vi "Actor Core.vi"(8 "error in":cluster{"状态":bool, "代码":i32, "源":string} caption="错误输入", 11 "Beta":refnum<class "Beta.lvclass"> caption="DNL_Beta") -> (0 "error out":cluster{"状态":bool, "代码":i32, "源":string} caption="错误输出", 3 "操作者输出":refnum<class "Actor.lvclass">)   [LabVIEW 2013, in "Beta操作者.lvlib" / "Beta.lvclass"]
doc: "Actor Core.vi包含操作者的主要消息处理循环。操作者通常位于该循环中，在各种消息到达时对消息进行处理。如Do.vi消息返回任何错误，该循环将停止运行，错误代码43将被作为“无错误停止”的标准信号发送给调用方。如需更改上述行为，可在子孙类的Handle Error.vi中对该部分逻辑进行重写。"
uses:
  Beta.lvclass
  <vilib>/ActorFramework/Actor/Actor.lvclass
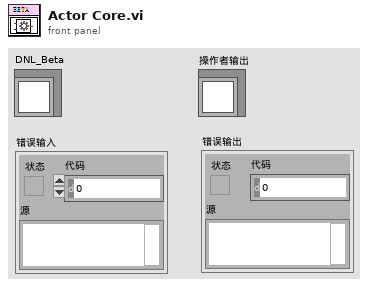
[diagram p1: front panel]
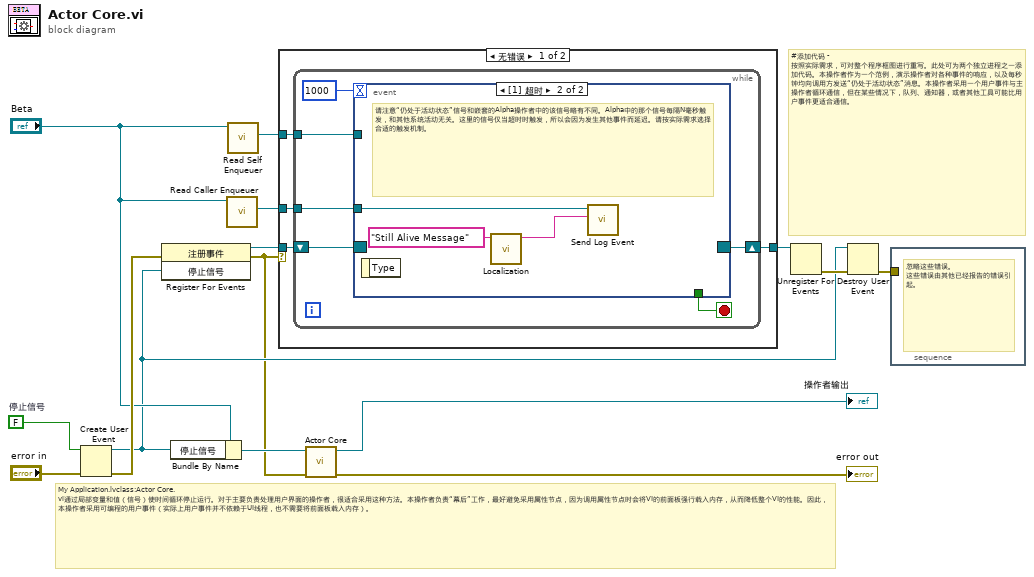
[diagram p0: block diagram]
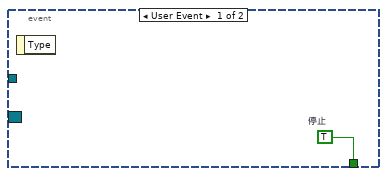
[diagram p2: hidden frame]
diagram:
  w11 = FALSE  # 停止信号
  # "My Application.lvclass:Actor Core.vi通过局部变量和值（信号）使时间循环停止运行。对于主要负责处理用户界面的操作者，很适合采用这种方法。本操作者负责“幕后”工作，最好避免采用属性节点，因为调用属性节点时会将VI的前面板强行载入内存，从而降低整个VI的性能。因此，本操作者采用可编程的用户事件（实际上用户事件并不依赖于UI线程，也不需要将前面板载入内存）。"
  # "#添加代码 - 按照实际需求，可对整个程序框图进行重写。此处可为两个独立进程之一添加代码。本操作者作为一个范例，演示操作者对各种事件的响应，以及每秒钟均向调用方发送“仍处于活动状态”消息。本操作者采用一个用户事件与主操作者循环通信，但在某些情况下，队列、通知器，或者其他工具可能比用户事件更适合通信。"
  n1 = Create User Event(user event datatype=w11, error in="error in") -> (user event=w4:refnum<user-event>, error out=w10:errorcluster)
  n2 = register-events(error in=w10, w4) -> (reference out=w9:refnum<event-registration>, error out=w2:errorcluster)  [unwired: 1 in]
  n3 = Bundle By Name(cluster="Beta", "停止信号"=w4) -> (w6:refnum<class "Beta.lvclass">)
  n4 = call <vilib>:"Read Caller Enqueuer.vi"("Actor"="Beta") -> ("Caller Enqueuer"=w13:refnum<class "Message Enqueuer.lvclass">)  [unwired: 10 in]
  n5 = call <vilib>:"Read Self Enqueuer.vi"("Actor"="Beta") -> ("Self Enqueuer"=w14:refnum<class "Message Enqueuer.lvclass">)  [unwired: 10 in]
  n6 = case shown="无错误" w2 {
    tunnel: w14 -> [w19 _]
    tunnel: w13 -> [w18 _]
    tunnel: w9 -> [w17 w30]
    tunnel: [w16 w30] -> w3
    frame No Error {
      n7 = while {
        tunnel: w19 -> [w24]
        tunnel: w18 -> [w23]
        shift-right: [w20] -> w16
        shift-left: w17 -> [w21]
        stop <- w25 stop-if-true
        n8 = event shown="[1] 超时" {
          selector: w21 -> [_ _]
          dyn-events: [_ _] -> w20
          timeout: 1000 -> [_ _]
          tunnel: [w26 _] -> w25
          tunnel: w24 -> [_ _]
          tunnel: w23 -> [_ w29]
          event User Event {
            w26 = TRUE  # 停止
            n9 = event-data() -> ()  [unwired: 1 in, 1 out]
          }
          event Timeout {
            # "请注意“仍处于活动状态”信号和嵌套的Alpha操作者中的该信号略有不同。Alpha中的那个信号每隔N毫秒触发，和其他系统活动无关。这里的信号仅当超时时触发，所以会因为发生其他事件而延迟。请按实际需求选择合适的触发机制。"
            n10 = event-data() -> ()  [unwired: 1 in, 1 out]
            n11 = call "Localization.vi"("未本地化"="Still Alive Message" ("Unlocalized")) -> ("本地化"=w27:string)  [unwired: 10 in]
            n12 = call "Send Log Event.vi"("事件文本"=w27, "消息待入队列"=w29) -> ()  [unwired: 9 in, 1 out]
          }
        }
      }
    }
    frame Error {
    }
  }
  n13 = call-parent "Actor Core.vi"("error in"=w2, "Actor in"=w6) -> ("error out"=→"error out":errorcluster, "Actor out"=→"操作者输出":refnum<class "Actor.lvclass">)  [unwired: 8 in]
  n14 = Unregister For Events(event registration refnum=w3) -> (error out=w5:errorcluster)  [unwired: 1 in]
  n15 = Destroy User Event(user event=w4, error in=w5) -> (error out=w1:errorcluster)
  n16 = stacked-sequence {
    tunnel: w1 -> [_]
    frame #0 {
      # "忽略这些错误。\n这些错误由其他已经报告的错误引起。"
    }
  }
